vi "T_S id.vi"() -> ()   [LabVIEW 2017, in "Konfiguracja.lvlib"]
uses:
  Libraries/Konfiguracja/Konfiguracja.lvlib
  GUI/Controls/ts selector.ctl
  <vilib>/Plasmionique/MB Master/MB_Master_Serial/MB_Master_Serial.lvclass
  D:/Program Files (x86)/National Instruments/LabVIEW 2017/vi.lib/Plasmionique/MB Master/MB_Master/MB_Master.lvclass
  <vilib>/Plasmionique/MB Master/MB Master.lvlib
panel:
  out "Undo term id":dbl=1.0 min=1.0 max=20.0 step=1.0
  out "Undo slave id":dbl=2.0 min=2.0 max=128.0 step=1.0
  out "Rejestry":u16[](array[numeric])
  in  "System Tab":enum32{"Page 1"}(tab)
  out "String id":string caption="Zapis nr id pomyślny?"
  out "String address":string caption="Zapis adresu pomyślny?"
  in  "VISA":refnum<visa-resource-name>
  in  "Save":bool
  in  "Docelowy nr id \nslave'a":dbl=2.0 min=2.0 max=127.0 step=1.0
  in  "Aktualny nr id \nslave'a":dbl=1.0 min=1.0 max=127.0 step=1.0
  in  "Undo":bool
  in  "Nr id termometru":dbl=1.0 min=1.0 max=20.0 step=1.0
  in  "Nr id slave'a":dbl=2.0 min=2.0 max=128.0 step=1.0
  in  "Copy":bool
  # "Należy wybrać nr id slave'a oraz termometru do którego \nma zostać skopiowany adres odczytany z termometru \npodłączonego do local 1-wire"
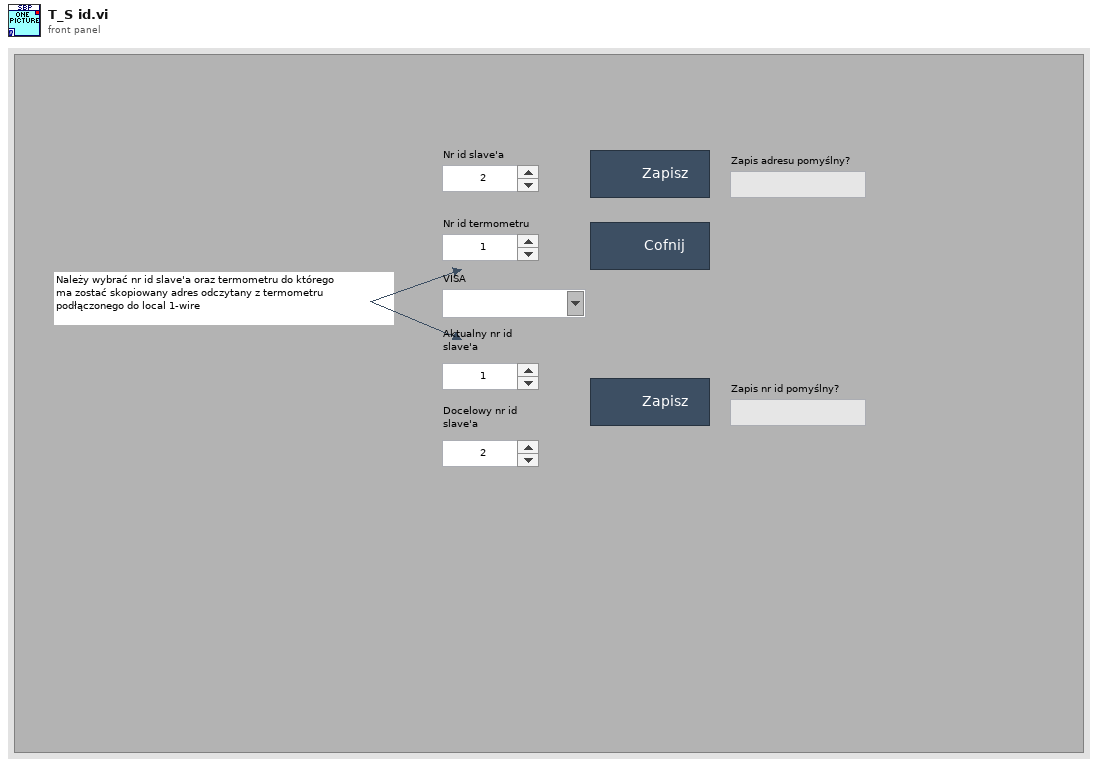
[diagram p1: front panel]
types:
  T1 = typedef "ts selector.ctl" = enum16{"undo", "wait for input", "adress", "id", "exit"}
  T2 = cluster{"baud rate (bps)":u32, "stop bits":u16, "parity":u16, "flow control":u16, "timeout":u32, "retries":i32}
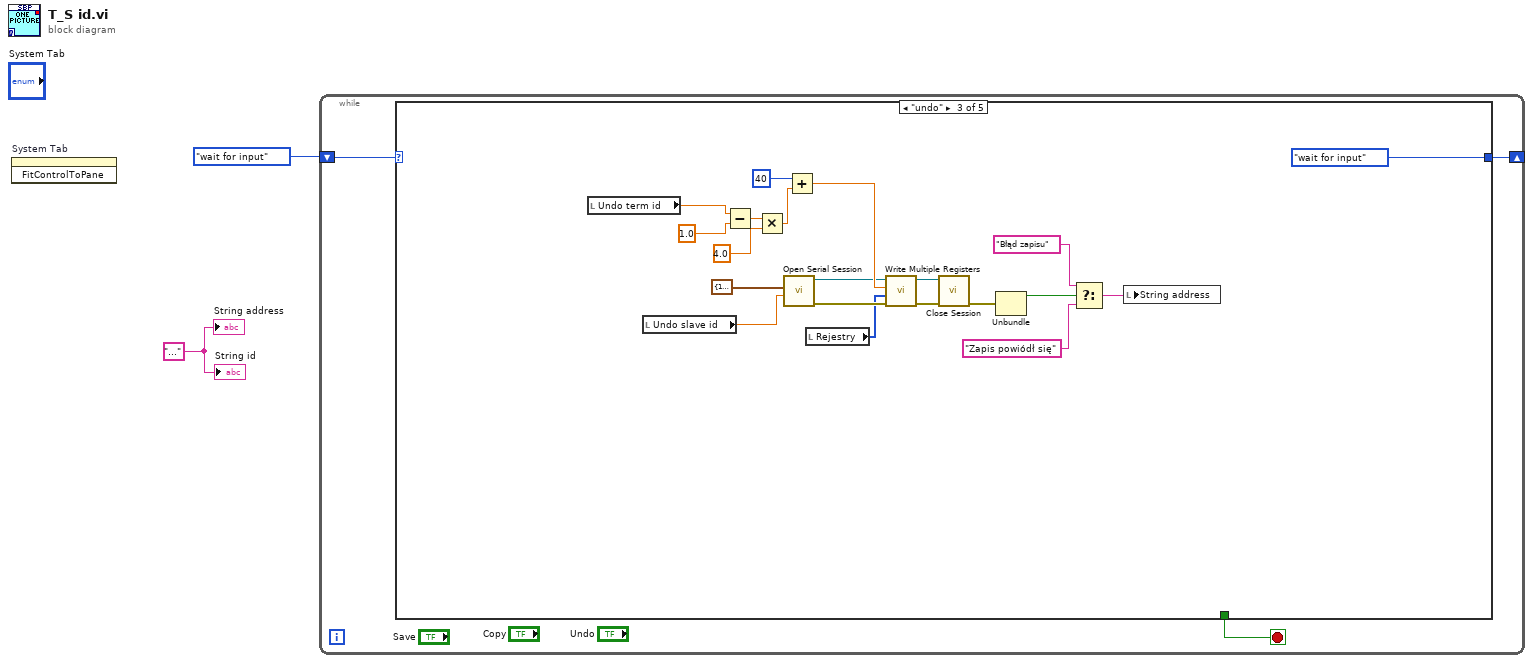
[diagram p0: block diagram]
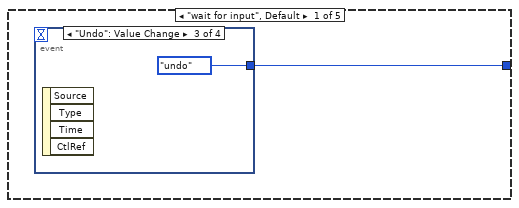
[diagram p2: hidden frame]
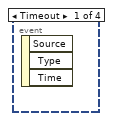
[diagram p3: hidden frame]
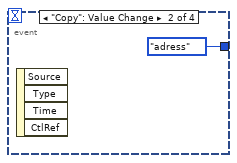
[diagram p4: hidden frame]
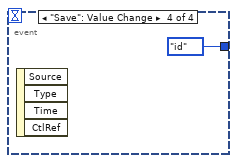
[diagram p5: hidden frame]
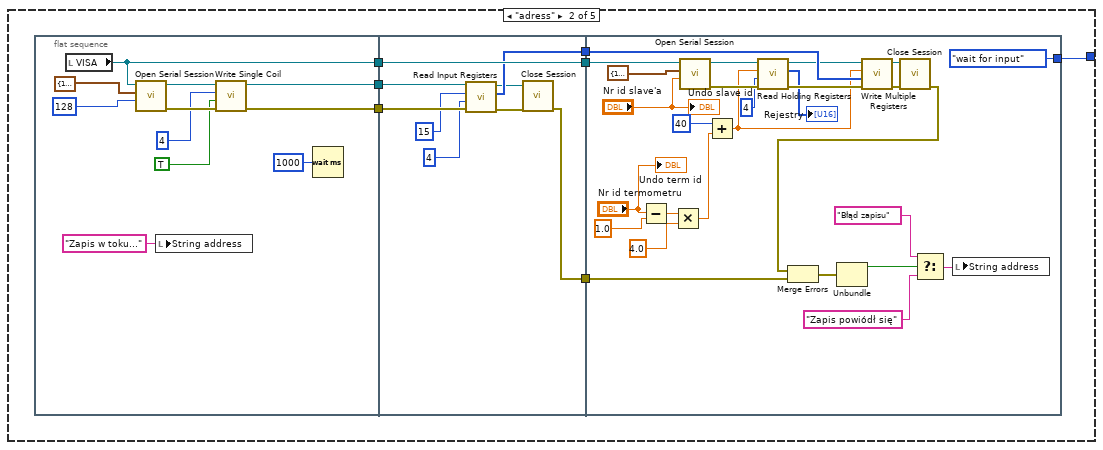
[diagram p6: hidden frame]
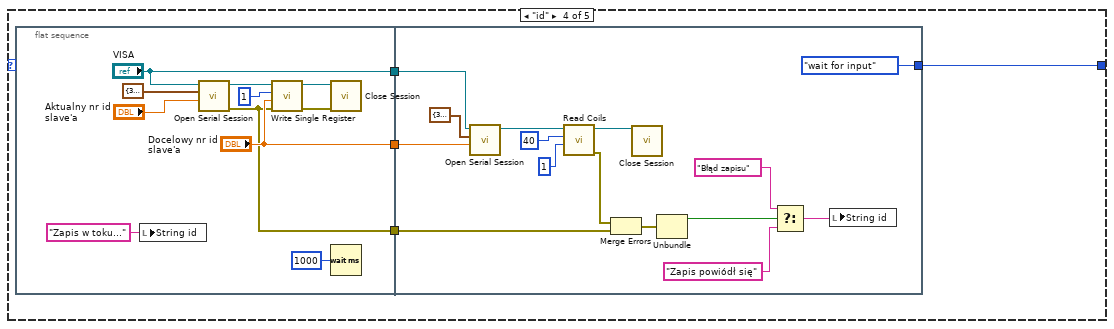
[diagram p7: hidden frame]
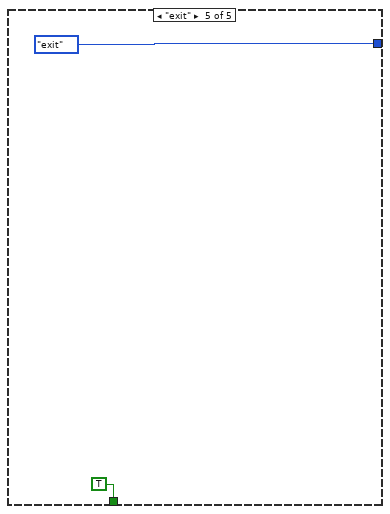
[diagram p8: hidden frame]
diagram:
  w1 = "..." ("String id")
  n1 = invoke on="System Tab" class="TabCtl (strict)" method="FitControlToPane"() -> ()  [unwired: 3 in, 3 out]
  n2 = while {
    shift-right: [w3] -> _
    shift-left: ts_selector."wait for input" -> [w4]
    stop <- w5 stop-if-true
    n3 = case shown="\"undo\"" w4 {
      tunnel: [_ _ _ _ TRUE] -> w5
      tunnel: [w6 w10 ts_selector."wait for input" w85 ts_selector."exit"] -> w3
      frame "wait for input", Default {
        n4 = event shown="[2] \"Undo\": Value Change" {
          selector: _ -> [_ _ _ _]
          dyn-events: _ -> [_ _ _ _]
          timeout: _ -> [_ _ _ _]
          tunnel: [_ ts_selector."adress" ts_selector."undo" ts_selector."id"] -> w6
          event Timeout {
            n5 = event-data() -> ()  [unwired: 1 in, 3 out]
          }
          event "Copy": Value Change {
            n6 = event-data() -> ()  [unwired: 1 in, 4 out]
          }
          event "Undo": Value Change {
            n7 = event-data() -> ()  [unwired: 1 in, 4 out]
          }
          event "Save": Value Change {
            n8 = event-data() -> ()  [unwired: 1 in, 4 out]
          }
        }
      }
      frame "adress" {
        n9 = flat-sequence {
          tunnel: [w25] -> w16
          tunnel: [w22] -> w13
          tunnel: [w21] -> w12
          tunnel: w16 -> [w36]
          tunnel: [w36] -> w15
          tunnel: [w31] -> w14
          tunnel: w13 -> [w34]
          tunnel: w12 -> [w35]
          tunnel: [w28] -> w11
          tunnel: w15 -> [w61]
          tunnel: w14 -> [w56]
          tunnel: w11 -> [w50]
          tunnel: [ts_selector."wait for input"] -> w10
          frame #0 {
            n10 = local read "VISA"() -> (w25:refnum<visa-resource-name>)
            n11 = call <vilib>:"Open Serial Session.vi"("Slave ID"=u8 128, "Serial Config"=T2 {"baud rate (bps)"=115200, "stop bits"=10, "parity"=0, "flow control"=0, "timeout"=1000, "retries"=1}, "VISA Resource"=w25) -> ("Error out"=w23:errorcluster, "MB_Serial session"=w24:refnum<class "MB_Master_Serial.lvclass">)  [unwired: 7 in]
            n12 = local write "String address"("Zapis w toku..." ("String address")) -> ()
            n13 = call <vilib>:"Write Single Coil.vi"("error in (no error)"=w23, "value"=TRUE, "address"=u16 4, "MB session in"=w24) -> ("error out"=w22:errorcluster, "MB session out"=w21:refnum<class "MB_Master_Serial.lvclass">)  [unwired: 6 in]
            n14 = Wait (ms)(milliseconds to wait=u32 1000) -> ()  [unwired: 1 out]
          }
          frame #1 {
            n15 = call <vilib>:"Read Input Registers.vi"("error in (no error)"=w34, "quantity"=u16 4, "starting address"=u16 15, "MB session in"=w35) -> ("error out"=w29:errorcluster, "Registers"=w31:u16[], "MB session out"=w30:refnum<class "MB_Master_Serial.lvclass">)  [unwired: 5 in]
            n16 = call-dynamic "Close Session.vi"("error in (no error)"=w29, "MB_Serial session"=w30) -> ("error out"=w28:errorcluster)  [unwired: 9 in]
          }
          frame #2 {
            n17 = Subtract(x="Nr id termometru", y=1.0) -> (x-y=w52:dbl)
            n18 = Multiply(x=w52, y=4.0) -> (x*y=w53:dbl)
            n19 = call <vilib>:"Open Serial Session.vi"("Slave ID"="Nr id slave'a", "Serial Config"=T2 {"baud rate (bps)"=115200, "stop bits"=10, "parity"=0, "flow control"=0, "timeout"=1000, "retries"=1}, "VISA Resource"=w61) -> ("Error out"=w42:errorcluster, "MB_Serial session"=w43:refnum<class "MB_Master_Serial.lvclass">)  [unwired: 7 in]
            n20 = Add(x=40, y=w53) -> (x+y=w41:dbl)
            n21 = call <vilib>:"Read Holding Registers.vi"("error in (no error)"=w42, "quantity"=u16 4, "starting address"=w41, "MB session in"=w43) -> ("error out"=w62:errorcluster, "Registers"=→"Rejestry":u16[], "MB session out"=w40:refnum<class "MB_Master_Serial.lvclass">)  [unwired: 5 in]
            n22 = call <vilib>:"Write Multiple Registers.vi"("error in (no error)"=w62, "values"=w56, "starting address"=w41, "MB session in"=w40) -> ("error out"=w55:errorcluster, "MB session out"=w54:refnum<class "MB_Master_Serial.lvclass">)  [unwired: 6 in]
            n23 = call-dynamic "Close Session.vi"("error in (no error)"=w55, "MB_Serial session"=w54) -> ("error out"=w37:errorcluster)  [unwired: 9 in]
            n24 = Merge Errors(w37, w50) -> (w49:errorcluster)
            n25 = Unbundle(w49) -> ("status"=w48:bool)  [unwired: 2 out]
            n26 = Select(t="Błąd zapisu" ("String address"), s=w48, f="Zapis powiódł się" ("String address")) -> (s? t:f=w45:string)
            n27 = local write "String address"(w45) -> ()
            "Undo slave id" <- "Nr id slave'a"
            "Undo term id" <- "Nr id termometru"
          }
        }
      }
      frame "undo" {
        n28 = local read "Undo term id"() -> (w68:dbl)
        n29 = local read "Undo slave id"() -> (w69:dbl)
        n30 = Subtract(x=w68, y=1.0) -> (x-y=w76:dbl)
        n31 = Multiply(x=w76, y=4.0) -> (x*y=w77:dbl)
        n32 = call <vilib>:"Open Serial Session.vi"("Slave ID"=w69, "Serial Config"=T2 {"baud rate (bps)"=115200, "stop bits"=10, "parity"=0, "flow control"=0, "timeout"=1000, "retries"=1}) -> ("Error out"=w65:errorcluster, "MB_Serial session"=w66:refnum<class "MB_Master_Serial.lvclass">)  [unwired: 8 in]
        n33 = Add(x=40, y=w77) -> (x+y=w70:dbl)
        n34 = local read "Rejestry"() -> (w64:u16[])
        n35 = call <vilib>:"Write Multiple Registers.vi"("error in (no error)"=w65, "values"=w64, "starting address"=w70, "MB session in"=w66) -> ("error out"=w79:errorcluster, "MB session out"=w78:refnum<class "MB_Master_Serial.lvclass">)  [unwired: 6 in]
        n36 = call-dynamic "Close Session.vi"("error in (no error)"=w79, "MB_Serial session"=w78) -> ("error out"=w67:errorcluster)  [unwired: 9 in]
        n37 = Unbundle(w67) -> ("status"=w74:bool)  [unwired: 2 out]
        n38 = Select(t="Błąd zapisu" ("String address"), s=w74, f="Zapis powiódł się" ("String address")) -> (s? t:f=w71:string)
        n39 = local write "String address"(w71) -> ()
      }
      frame "id" {
        n40 = flat-sequence {
          tunnel: ["Docelowy nr id \nslave'a"] -> w87
          tunnel: ["VISA"] -> w86
          tunnel: [w91] -> w84
          tunnel: w87 -> [w113]
          tunnel: w86 -> [w111]
          tunnel: [ts_selector."wait for input"] -> w85
          tunnel: w84 -> [w104]
          frame #0 {
            n41 = local write "String id"("Zapis w toku..." ("String id")) -> ()
            n42 = call <vilib>:"Open Serial Session.vi"("Slave ID"="Aktualny nr id \nslave'a", "Serial Config"=T2 {"baud rate (bps)"=38400, "stop bits"=10, "parity"=0, "flow control"=0, "timeout"=1000, "retries"=1}, "VISA Resource"="VISA") -> ("Error out"=w91:errorcluster, "MB_Serial session"=w96:refnum<class "MB_Master_Serial.lvclass">)  [unwired: 7 in]
            n43 = call <vilib>:"Write Single Register.vi"("error in (no error)"=w91, "value"="Docelowy nr id \nslave'a", "address"=u16 1, "MB session in"=w96) -> ("error out"=w89:errorcluster, "MB session out"=w94:refnum<class "MB_Master_Serial.lvclass">)  [unwired: 6 in]
            n44 = call-dynamic "Close Session.vi"("error in (no error)"=w89, "MB_Serial session"=w94) -> ()  [unwired: 9 in, 1 out]
            n45 = Wait (ms)(milliseconds to wait=u32 1000) -> ()  [unwired: 1 out]
          }
          frame #1 {
            n46 = call <vilib>:"Open Serial Session.vi"("Slave ID"=w113, "Serial Config"=T2 {"baud rate (bps)"=38400, "stop bits"=10, "parity"=0, "flow control"=0, "timeout"=1000, "retries"=1}, "VISA Resource"=w111) -> ("MB_Serial session"=w108:refnum<class "MB_Master_Serial.lvclass">)  [unwired: 7 in, 1 out]
            n47 = call <vilib>:"Read Coils.vi"("quantity"=u16 1, "starting address"=u16 40, "MB session in"=w108) -> ("error out"=w105:errorcluster, "MB session out"=w109:refnum<class "MB_Master_Serial.lvclass">)  [unwired: 6 in, 1 out]
            n48 = Merge Errors(w105, w104) -> (w103:errorcluster)
            n49 = call-dynamic "Close Session.vi"("MB_Serial session"=w109) -> ()  [unwired: 10 in, 1 out]
            n50 = Unbundle(w103) -> ("status"=w100:bool)  [unwired: 2 out]
            n51 = Select(t="Błąd zapisu" ("String address"), s=w100, f="Zapis powiódł się" ("String address")) -> (s? t:f=w99:string)
            n52 = local write "String id"(w99) -> ()
          }
        }
      }
      frame "exit" {
      }
    }
  }
  "String address" <- w1
  "String id" <- w1
